vi "Stop.vi"(8 "error in":errorcluster, 11 "reference in":refnum<class "Instrument.lvclass">) -> (0 "error out":errorcluster, 3 "reference out":refnum<class "Instrument.lvclass">)   [LabVIEW 2023, in "HAL GOOP4.lvlib" / "Instrument.lvclass"]
uses:
  Instrument.lvclass
  Interfaces/IConfigure/IConfigure.lvclass
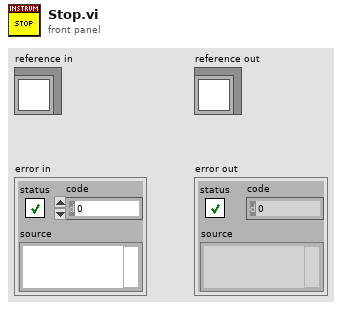
[diagram p1: front panel]
types:
  T1 = typedef "HAL GOOP4.lvlib/Instrument.lvclass/ObjectAttributes.ctl" = cluster{"IConfigure":refnum<class "IConfigure.lvclass">, "Ref Count":i16, "Start Count":i16}
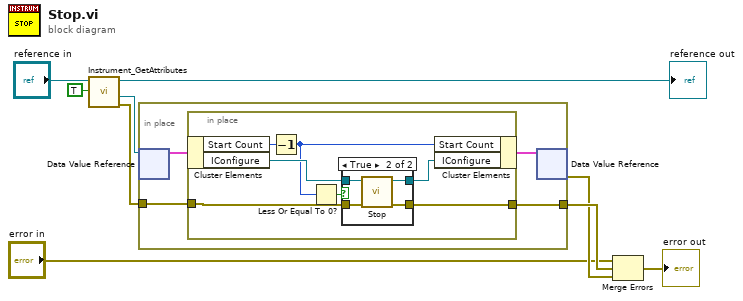
[diagram p0: block diagram]
diagram:
  n1 = call "Instrument_GetAttributes.vi"("OnlyGetDvrReference(False)"=TRUE, "reference in"="reference in") -> ("Error Out"=w8:errorcluster, "DataRef"=w9:refnum<data-value>, "reference out"=→"reference out":refnum<class "Instrument.lvclass">)  [unwired: 6 in, 1 out]
  n2 = in-place {
    in-place-border: w8 -> [w11]
    in-place-border: [w10] -> w4
    n3 = in-place-dvr #1(w9) -> (w13:T1)  [unwired: 1 out]
    n4 = in-place {
      in-place-border: w11 -> [w18]
      in-place-border: [w17] -> w10
      n5 = in-place-cluster #2(w13) -> ("Start Count"=w16:i16, "IConfigure"=w20:refnum<class "IConfigure.lvclass">)
      n6 = Decrement(x=w16) -> (x-1=w15:i16)
      n7 = Less Or Equal To 0?(x=w15) -> (x <= 0?=w14:bool)
      n8 = case shown="True" w14 {
        tunnel: w20 -> [w21 w26]
        tunnel: [w21 w25] -> w19
        tunnel: w18 -> [w22 w24]
        tunnel: [w22 w23] -> w17
        frame False {
        }
        frame True {
          n9 = call-dynamic "Stop.vi"("error in (no error)"=w24, "IConfigure in"=w26) -> ("error out"=w23:errorcluster, "IConfigure out"=w25:refnum<class "IConfigure.lvclass">)  [unwired: 8 in]
        }
      }
      n10 = in-place-cluster #2("Start Count"=w15, "IConfigure"=w19) -> (w12:T1)
    }
    n11 = in-place-dvr #1(w12) -> (w3:errorcluster)  [unwired: 1 out]
  }
  n12 = Merge Errors("error in", w4, w3) -> (→"error out":errorcluster)
